vi "8-bit video export-setup.vi"(11 "selected AVI file path":path) -> (1 "output cluster":T2, 3 "cancelled":bool)   [LabVIEW 2013]
uses:
  <vilib>/vision/Avi.llb/IMAQ AVI2 Refnum.ctl
  Globals/gl_Time series viewer globals.vi
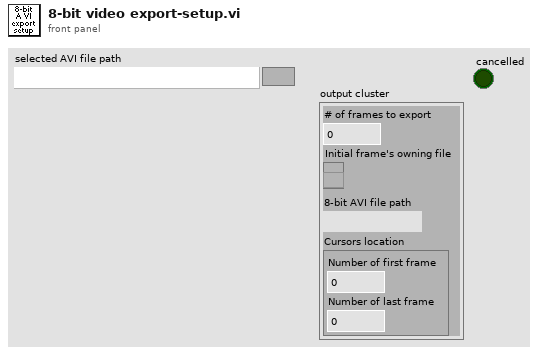
[diagram p1: front panel]
types:
  T1 = typedef "IMAQ AVI2 Refnum.ctl" = refnum<k20>
  T2 = cluster{"# of frames to export":i32, "Initial frame's owning file":T1, "8-bit AVI file path":path, "Cursors location":cluster{"Number of first frame":i32, "Number of last frame":i32}}
  T3 = enum16{"Export from full dataset", "Export from cursors selection"}
  T4 = cluster{"Number of first frame":i32, "Number of last frame":i32}
  T5 = cluster{"Caption-Right button":string, "Caption-Left button":string, "Message to display":string, "Delay before close":u32, "Window Colour":u32, "Cancel button disabled?":enum8{"Enabled", "Disabled", "Disabled and Grayed Out"}}
  T6 = typedef "AVI modes refs cluster.ctl" = cluster{"AVI1 ref":T7, "AVI2 refs":T1[], "AVI # frames":u32[]}
  T7 = typedef "AviRefnum.ctl" = refnum<k1>
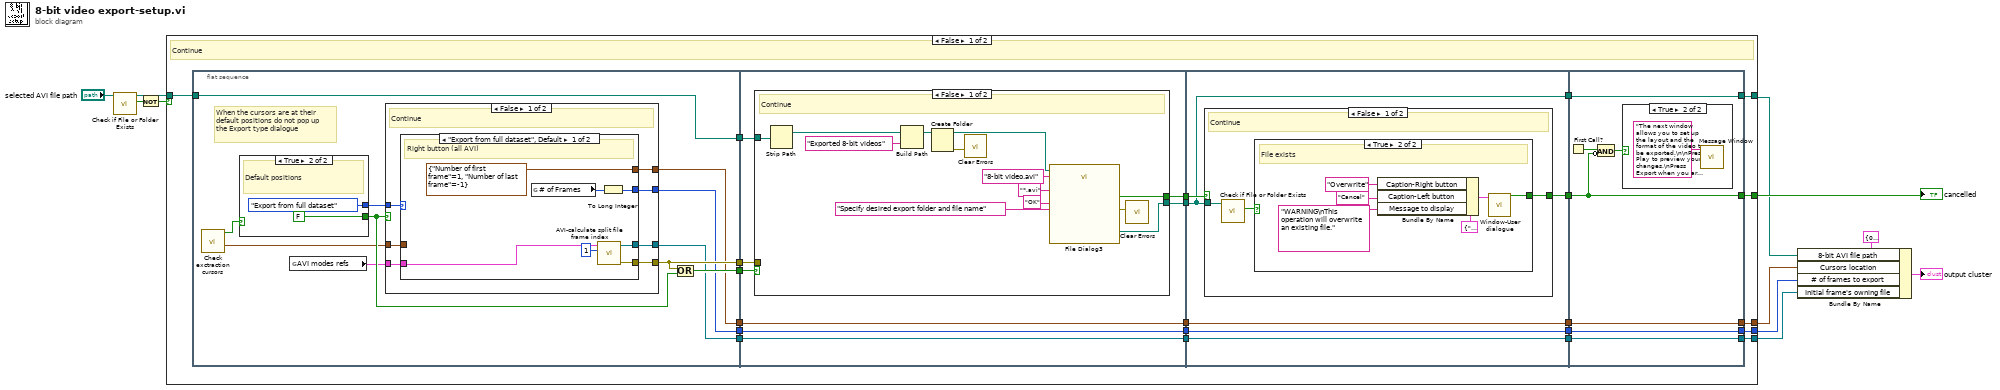
[diagram p0: block diagram]
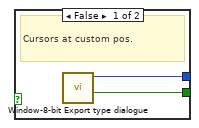
[diagram p2: hidden frame]
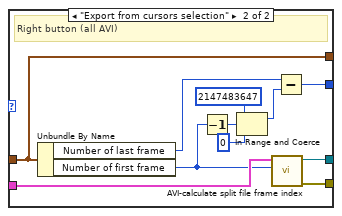
[diagram p3: hidden frame]
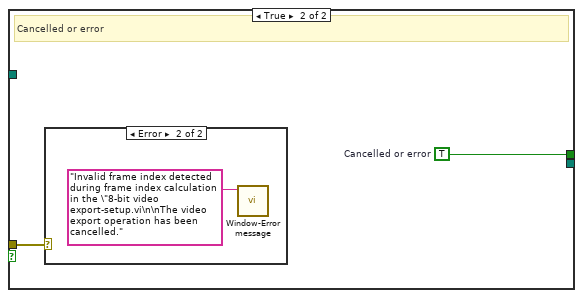
[diagram p5: hidden frame]
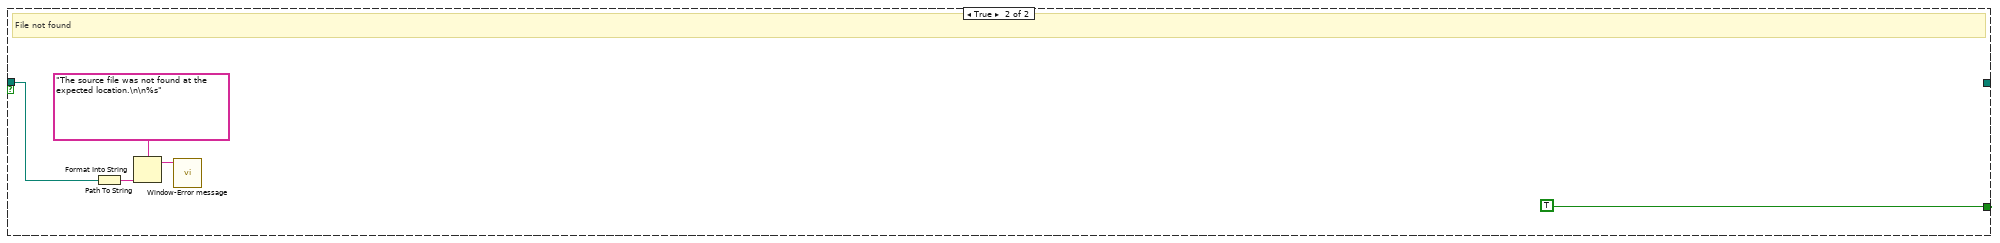
[diagram p10: hidden frame]
diagram:
  n1 = call <vilib>:"Check if File or Folder Exists.vi"("path"="selected AVI file path") -> ("file or folder exists?"=w1:bool, "dup path"=w10:path)  [unwired: 8 in, 1 out]
  n2 = Not(x=w1) -> (.not. x?=w9:bool)
  n3 = case shown="False" w9 {
    tunnel: [w31 _] -> w5
    tunnel: [w30 TRUE ("cancelled")] -> w6
    tunnel: w10 -> [w29 w122]
    tunnel: [w19 _] -> w4
    tunnel: [w18 _] -> w3
    tunnel: [w17 _] -> w2
    frame False {
      # "Continue"
      n4 = flat-sequence {
        tunnel: [w43] -> w33
        tunnel: w29 -> [w43]
        tunnel: [w41] -> w27
        tunnel: [w40] -> w26
        tunnel: [w39] -> w24
        tunnel: [w38] -> w23
        tunnel: [w37] -> w21
        tunnel: w33 -> [w81]
        tunnel: [w80] -> w32
        tunnel: [w79] -> w28
        tunnel: w27 -> [w78]
        tunnel: w26 -> [w77]
        tunnel: [w76] -> w25
        tunnel: w24 -> [w76]
        tunnel: w23 -> [w75]
        tunnel: [w75] -> w22
        tunnel: w21 -> [w74]
        tunnel: [w74] -> w20
        tunnel: w32 -> [w103]
        tunnel: w28 -> [w98]
        tunnel: w25 -> [w100]
        tunnel: w22 -> [w99]
        tunnel: w20 -> [w101]
        tunnel: [w98] -> w16
        tunnel: [w102] -> w15
        tunnel: [w101] -> w14
        tunnel: [w100] -> w13
        tunnel: [w99] -> w12
        tunnel: [w117] -> w17
        tunnel: [w118] -> w18
        tunnel: [w119] -> w19
        tunnel: [w115] -> w30
        tunnel: [w120] -> w31
        tunnel: w16 -> [w120]
        tunnel: w15 -> [w115]
        tunnel: w14 -> [w119]
        tunnel: w13 -> [w118]
        tunnel: w12 -> [w117]
        frame #0 {
          # "When the cursors are at their default positions do not pop up the Export type dialogue"
          n5 = call "Check exctraction cursors.vi"() -> ("Cursors positions"=w36:T4, "Extraction cursors at default positions"=w35:bool)  [unwired: 9 in, 1 out]
          n6 = case shown="True" w35 {
            tunnel: [w46 T3."Export from full dataset" ("Export type")] -> w44
            tunnel: [w45 FALSE ("Cancelled")] -> w42
            frame False {
              # "Cursors at custom pos."
              n7 = call "Window-8-bit Export type dialogue.vi"() -> ("Cancelled"=w45:bool, "Export type"=w46:T3)  [unwired: 10 in]
            }
            frame True {
              # "Default positions"
            }
          }
          n8 = global read "gl_Time series viewer globals.vi" "AVI modes refs"() -> (w34:T6)
          n9 = case shown="False" w42 {
            tunnel: w44 -> [w55 _]
            tunnel: [w54 _] -> w37
            tunnel: [w50 _] -> w39
            tunnel: w34 -> [w53 _]
            tunnel: [w52 _] -> w40
            tunnel: [w51 _] -> w38
            tunnel: w36 -> [w49 _]
            frame False {
              # "Continue"
              n10 = case shown="\"Export from full dataset\", Default" w55 {
                tunnel: [w57 w71] -> w50
                tunnel: [w61 w72] -> w54
                tunnel: w53 -> [w56 w73]
                tunnel: [w59 w66] -> w52
                tunnel: [T4 {"Number of first frame"=1, "Number of last frame"=-1} ("Cursors location") w63] -> w51
                tunnel: w49 -> [_ w63]
                frame "Export from full dataset", Default {
                  # "Right button (all AVI)"
                  n11 = global read "gl_Time series viewer globals.vi" "# of Frames"() -> (w62:u32)
                  n12 = call "AVI-calculate split file frame index.vi"("Frame number (unity-based) in"=1, "AVI modes refs"=w56) -> ("error out"=w59:errorcluster, "AVI2 split file ref"=w61:T1)  [unwired: 6 in, 2 out]
                  n13 = To Long Integer(number=w62) -> (32bit integer=w57:i32)
                }
                frame "Export from cursors selection" {
                  # "Right button (all AVI)"
                  n14 = Unbundle By Name(w63) -> ("Number of last frame"=w65:i32, "Number of first frame"=w64:i32)
                  n15 = Decrement(x=w64) -> (x-1=w70:i32)
                  n16 = In Range and Coerce(upper limit=2147483647, x=w70, lower limit=0) -> (coerced(x)=w67:i32)  [unwired: 1 out]
                  n17 = call "AVI-calculate split file frame index.vi"("Frame number (unity-based) in"=w64, "AVI modes refs"=w73) -> ("error out"=w66:errorcluster, "AVI2 split file ref"=w72:T1)  [unwired: 6 in, 2 out]
                  n18 = Subtract(x=w65, y=w67) -> (x-y=w71:i32)
                }
              }
            }
            frame True {
              # "Cancelled"
            }
          }
          n19 = Compound Arithmetic op=OR(w40, w42) -> (w41:bool)
        }
        frame #1 {
          n20 = case shown="False" w78 {
            tunnel: w81 -> [w94 _]
            tunnel: [w93 w96] -> w80
            tunnel: [w92 _] -> w79
            tunnel: w77 -> [_ w95]
            frame False {
              # "Continue"
              n21 = Strip Path(path=w94) -> (stripped path=w86:path)  [unwired: 1 out]
              n22 = Build Path(base path=w86, name or relative path="Exported 8-bit videos") -> (appended path=w84:path)
              n23 = Create Folder(path (use dialog)=w84) -> (created path=w83:path, error out=w82:errorcluster)  [unwired: 2 in, 1 out]
              n24 = call <vilib>:"Clear Errors.vi"("error in (no error)"=w82) -> ()  [unwired: 6 in, 1 out]
              n25 = call "File Dialog3"("start path"=w83, "prompt"="Specify desired export folder and file name" ("default name"), "button label"="OK", "default name"="8-bit video.avi", "pattern (all files)"="*.avi" ("pattern label")) -> ("selected path"=w92:path, "cancelled"=w93:bool, "error out"=w91:errorcluster)  [unwired: 7 in, 1 out]
              n26 = call <vilib>:"Clear Errors.vi"("error in (no error)"=w91) -> ()  [unwired: 6 in, 1 out]
            }
            frame True {
              w96 = TRUE  # Cancelled or error
              # "Cancelled or error"
              n27 = case shown="Error" w95 {
                frame No Error {
                }
                frame Error {
                  n28 = call "Window-Error message.vi"("Message"="Invalid frame index detected during frame index calculation in the \"8-bit video export-setup.vi\n\nThe video export operation has been cancelled.") -> ()  [unwired: 10 in, 1 out]
                }
              }
            }
          }
        }
        frame #2 {
          n29 = case shown="False" w103 {
            selector: w103 -> [_ w113]
            tunnel: w98 -> [w106 _]
            tunnel: [w104 w113] -> w102
            frame False {
              # "Continue"
              n30 = call <vilib>:"Check if File or Folder Exists.vi"("path"=w106) -> ("file or folder exists?"=w105:bool)  [unwired: 8 in, 2 out]
              n31 = case shown="True" w105 {
                tunnel: [_ w112] -> w104
                frame False {
                  # "File does not exist"
                }
                frame True {
                  # "File exists"
                  n32 = Bundle By Name(cluster=T5 {"Caption-Right button"="", "Caption-Left button"="", "Message to display"="", "Delay before close"=0, "Window Colour"=16448250, "Cancel button disabled?"=enum."Enabled"} ("Input cluster"), "Caption-Right button"="Overwrite" ("T button name (\"OK\")"), "Caption-Left button"="Cancel" ("F button name (\"Cancel\")"), "Message to display"="WARNING\nThis operation will overwrite an existing file." ("Message string")) -> (w109:T5)
                  n33 = call "Window-User dialogue.vi"("Input cluster"=w109) -> ("Left Button (Cancel)"=w112:bool)  [unwired: 10 in]
                }
              }
            }
            frame True {
              # "Cancelled"
            }
          }
        }
        frame #3 {
          n34 = First Call?() -> (First Call?: T/F=w116:bool)
          n35 = Compound Arithmetic op=AND(w116, invert w115) -> (w114:bool)
          n36 = case shown="True" w114 {
            frame False {
            }
            frame True {
              n37 = call "Message Window.vi"("Message string"="The next window allows you to set up the layout and the format of the video to be exported.\n\nPress Play to preview your changes.\nPress Export when you are done." ("Message to display")) -> ()  [unwired: 10 in, 1 out]
            }
          }
        }
      }
    }
    frame True {
      # "File not found"
      n38 = Path To String(path=w122) -> (string=w124:string)
      n39 = Format Into String(format string="The source file was not found at the expected location.\n\n%s", w124) -> (resulting string=w123:string)  [unwired: 2 in, 1 out]
      n40 = call "Window-Error message.vi"("Message"=w123) -> ()  [unwired: 10 in, 1 out]
    }
  }
  "cancelled" <- w6
  n41 = Bundle By Name(cluster=T2 {"# of frames to export"=0, "Initial frame's owning file"=refnum, "8-bit AVI file path"=path "", "Cursors location"={"Number of first frame"=0, "Number of last frame"=0}} ("output cluster"), "8-bit AVI file path"=w5, "Cursors location"=w2, "# of frames to export"=w3, "Initial frame's owning file"=w4) -> (→"output cluster":T2)
